vi "Change Name.vi"(8 "error in (no error)":errorcluster, 10 "New #":u16, 11 "Node Ptr":T1 format="%.0x") -> (0 "error out":errorcluster, 3 "Node Ptr out":T1 format="%.0x")   [LabVIEW 2011, in "PXIe-433x Custom Device.lvlib"]
uses:
  PXIe-433x Custom Device.lvlib
  <vilib>/NI Veristand/Custom Device API/Custom Device Item Ref.ctl
  Global.vi
  <vilib>/NI Veristand/Custom Device API/Get Item Property (U16).vi
  <vilib>/NI Veristand/Custom Device API/Custom Device API.lvlib
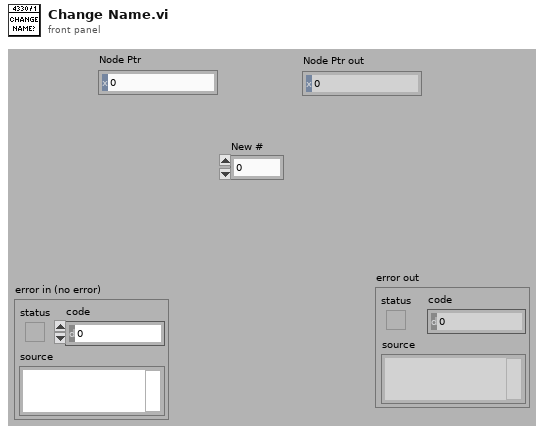
[diagram p1: front panel]
types:
  T1 = typedef "Custom Device API.lvlib/Custom Device Item Ref.ctl" = u64
  T2 = typedef "Custom Device API.lvlib/Custom Device Item Info.ctl" = cluster{"Name":string, "Is Channel":bool, "GUID":string}
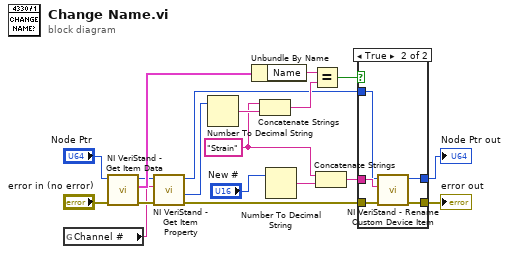
[diagram p0: block diagram]
diagram:
  w9 = "Strain" ("string")
  n1 = global read "Global.vi" "Channel #"() -> (w1:string)
  n2 = call <vilib>:"NI VeriStand - Get Item Data.vi"("error in (no error)"="error in (no error)", "Item Ref in"="Node Ptr") -> ("error out"=w16:errorcluster, "Item Info"=w18:T2, "Item Ref out"=w15:T1)  [unwired: 7 out]
  n3 = call-poly <vilib>:"NI VeriStand - Get Item Property.vi"("error in (no error)"=w16, "Property Name"=w1, "Item Ref in"=w15) -> ("error out"=w10:errorcluster, "Value"=w14:u16, "Item Ref out"=w5:T1)  [unwired: 5 in, 1 out]
  n4 = Number To Decimal String(number=w14) -> (decimal integer string=w13:string)  [unwired: 1 in]
  n5 = Unbundle By Name(w18) -> ("Name"=w12:string)
  n6 = Concatenate Strings(w9, w13) -> (w11:string)
  n7 = Number To Decimal String(number="New #") -> (decimal integer string=w7:string)  [unwired: 1 in]
  n8 = Equal?(x=w12, y=w11) -> (x = y?=w2:bool)
  n9 = Concatenate Strings(w9, w7) -> (w6:string)
  n10 = case shown="True" w2 {
    tunnel: w10 -> [w21 w26]
    tunnel: w6 -> [_ w25]
    tunnel: w5 -> [w20 w24]
    tunnel: [w20 w23] -> w4
    tunnel: [w21 w22] -> w3
    frame False {
    }
    frame True {
      n11 = call <vilib>:"NI VeriStand - Rename Custom Device Item.vi"("error in (no error)"=w26, "New Name"=w25, "Item Ref in"=w24) -> ("error out"=w22:errorcluster, "Item Ref out"=w23:T1)  [unwired: 7 out]
    }
  }
  "error out" <- w3
  "Node Ptr out" <- w4
